vi "Handle SET.vi"(8 "error in (no error)":errorcluster, 9 "data":variant, 10 "parameter":string, 11 "Instrument in":refnum<class "Instrument.lvclass">) -> (0 "error out":errorcluster, 2 "data out":variant, 3 "Instrument out":refnum<class "Instrument.lvclass">)   [LabVIEW 2019, in "Instrument.lvlib" / "Instrument.lvclass"]
uses:
  Instrument.lvclass
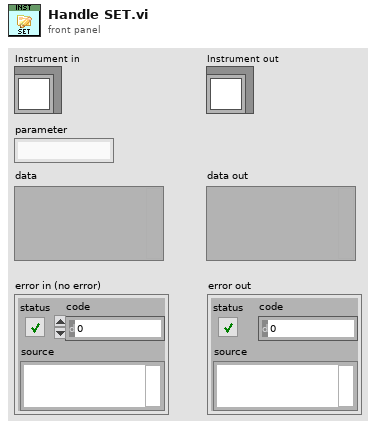
[diagram p1: front panel]
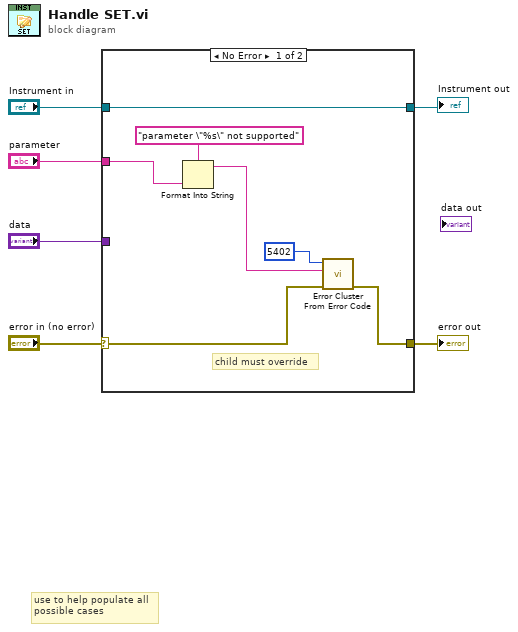
[diagram p0: block diagram]
diagram:
  # "use to help populate all\npossible cases"
  n1 = case shown="No Error" "error in (no error)" {
    selector: "error in (no error)" -> [w9 w14]
    tunnel: [w13 w15] -> w6
    tunnel: "Instrument in" -> [w13 w15]
    tunnel: [w8 w14] -> w4
    tunnel: "parameter" -> [w7 _]
    tunnel: "data" -> [_ _]
    frame No Error {
      # "child must override"
      n2 = Format Into String(format string="parameter \"%s\" not supported" ("error message (\"\")"), w7) -> (resulting string=w10:string)  [unwired: 2 in, 1 out]
      n3 = call <vilib>:"Error Cluster From Error Code.vi"("error in (no error)"=w9, "error message (\"\")"=w10, "error code (0)"=5402) -> ("error out"=w8:errorcluster)  [unwired: 6 in]
    }
    frame Error {
    }
  }
  "Instrument out" <- w6
  "error out" <- w4
